vi "Change_state.vi"(7 "connect (T)":bool=TRUE, 10 "Z_HSwitch_state in":T2={"Write"=FALSE, "Z1_ind visu"=5, "Z1_ind_blinking"=FALSE, "Z_HSwitch_out"=FALSE, "Z_HSwitch_visible"=FALSE, "Z_HSwitch_disabled"=enum."Enabled"}, 11 "Z_Source":T1=enum."local disabled") -> (1 "reset_timer":bool, 2 "Z_HSwitch_state out":T2, 3 "Z1_ind_state":T3 items=["init", "not connect", "local disabled", "local hand", "set hand", "hand", "set auto", "auto", "dist"], 4 "load_timer":bool)   [LabVIEW 2019, in "Heating.lvlib"]
uses:
  Heating.lvlib
  ctl/Z_Hswitch/AutoButton_state.ctl
  ctl/Z_source.ctl
  ctl/Z_Hswitch/Z_Hswitch.xctl
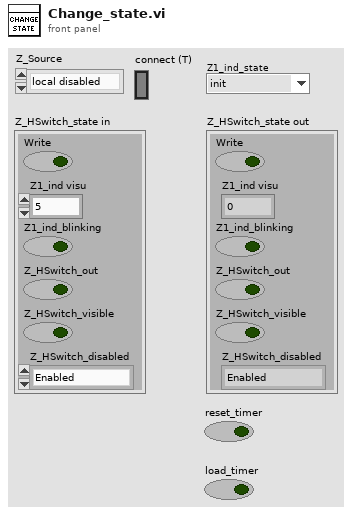
[diagram p1: front panel]
types:
  T1 = typedef "Heating.lvlib/Z_source.ctl" = enum8{"initialize", "local disabled", "local hand", "hand", "auto", "dist"}
  T2 = cluster{"Write":bool, "Z1_ind visu":u8, "Z1_ind_blinking":bool, "Z_HSwitch_out":bool, "Z_HSwitch_visible":bool, "Z_HSwitch_disabled":enum8{"Enabled", "Disabled", "Disabled and Grayed Out"}}
  T3 = typedef "Heating.lvlib/Z_Hswitch.xctl/AutoButton_state.ctl" = u16
  T4 = enum8{"Enabled", "Disabled", "Disabled and Grayed Out"}
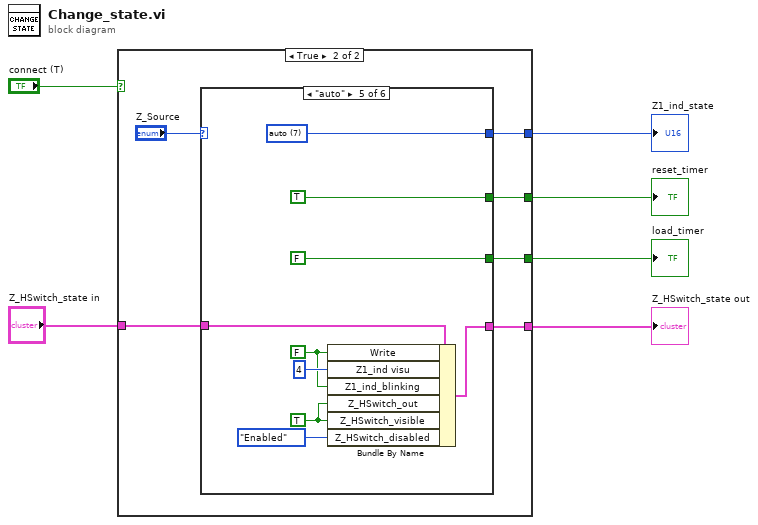
[diagram p0: block diagram]
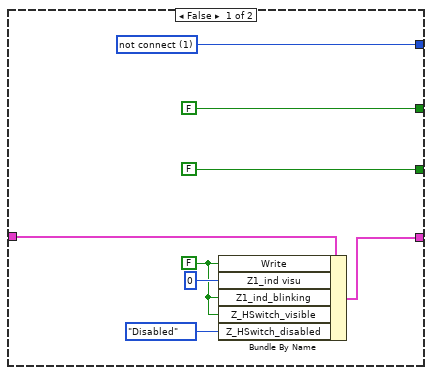
[diagram p2: hidden frame]
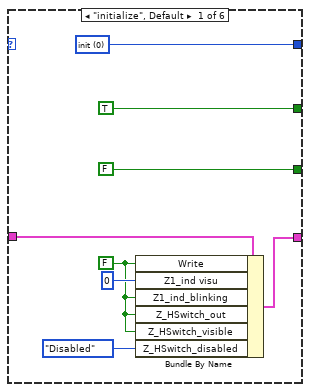
[diagram p3: hidden frame]
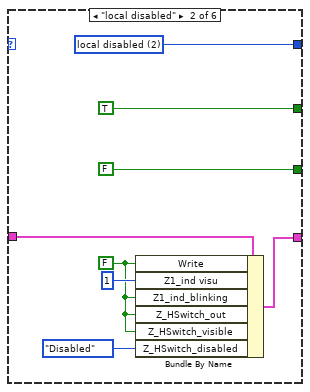
[diagram p4: hidden frame]
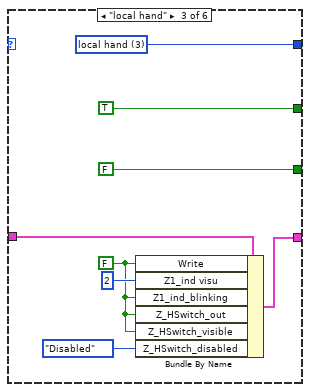
[diagram p5: hidden frame]
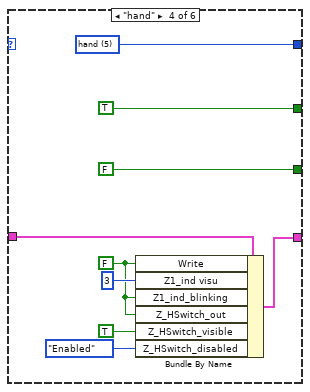
[diagram p6: hidden frame]
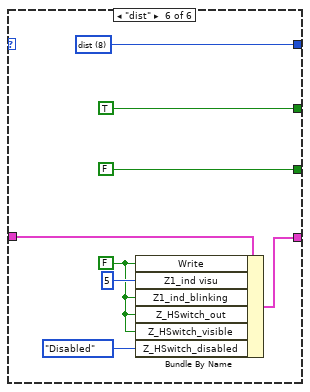
[diagram p7: hidden frame]
diagram:
  n1 = case shown="True" "connect (T)" {
    tunnel: "Z_HSwitch_state in" -> [w10 w20]
    tunnel: [w14 w18] -> w5
    tunnel: [FALSE ("Z_ASwitch") w17] -> w4
    tunnel: [FALSE ("Z_ASwitch") w16] -> w3
    tunnel: [w11 w15] -> w2
    frame False {
      w8 = FALSE ("Z_ASwitch")
      w14 = T3 1 items=["init", "not connect", "local disabled", "local hand", "set hand", "hand", "set auto", "auto", "dist"] ("Z1_State")
      n2 = Bundle By Name(cluster=w10, "Write"=w8, "Z1_ind visu"=u8 0, "Z1_ind_blinking"=w8, "Z_HSwitch_visible"=w8, "Z_HSwitch_disabled"=T4."Disabled" ("Disabled")) -> (w11:T2)
    }
    frame True {
      n3 = case shown="\"auto\"" "Z_Source" {
        tunnel: w20 -> [w26 w34 w42 w51 w60 w68]
        tunnel: [w25 w33 w41 w50 w59 w67] -> w18
        tunnel: [TRUE ("Z_ASwitch") TRUE ("Z_ASwitch") TRUE ("Z_ASwitch") TRUE ("Z_ASwitch") TRUE ("Z_ASwitch") TRUE ("Z_ASwitch")] -> w17
        tunnel: [FALSE ("Z_ASwitch") FALSE ("Z_ASwitch") FALSE ("Z_ASwitch") FALSE ("Z_ASwitch") FALSE ("Z_ASwitch") FALSE ("Z_ASwitch")] -> w16
        tunnel: [w22 w30 w38 w47 w56 w64] -> w15
        frame "initialize", Default {
          w21 = FALSE ("Z_ASwitch")
          w25 = T3 0 items=["init", "not connect", "local disabled", "local hand", "set hand", "hand", "set auto", "auto", "dist"] ("Z1_State")
          n4 = Bundle By Name(cluster=w26, "Write"=w21, "Z1_ind visu"=u8 0, "Z1_ind_blinking"=w21, "Z_HSwitch_out"=w21, "Z_HSwitch_visible"=w21, "Z_HSwitch_disabled"=T4."Disabled" ("Disabled")) -> (w22:T2)
        }
        frame "local disabled" {
          w29 = FALSE ("Z_ASwitch")
          w33 = T3 2 items=["init", "not connect", "local disabled", "local hand", "set hand", "hand", "set auto", "auto", "dist"] ("Z1_State")
          n5 = Bundle By Name(cluster=w34, "Write"=w29, "Z1_ind visu"=u8 1, "Z1_ind_blinking"=w29, "Z_HSwitch_out"=w29, "Z_HSwitch_visible"=w29, "Z_HSwitch_disabled"=T4."Disabled" ("Disabled")) -> (w30:T2)
        }
        frame "local hand" {
          w37 = FALSE ("Z_ASwitch")
          w41 = T3 3 items=["init", "not connect", "local disabled", "local hand", "set hand", "hand", "set auto", "auto", "dist"] ("Z1_State")
          n6 = Bundle By Name(cluster=w42, "Write"=w37, "Z1_ind visu"=u8 2, "Z1_ind_blinking"=w37, "Z_HSwitch_out"=w37, "Z_HSwitch_visible"=w37, "Z_HSwitch_disabled"=T4."Disabled" ("Disabled")) -> (w38:T2)
        }
        frame "hand" {
          w46 = FALSE ("Z_ASwitch")
          w50 = T3 5 items=["init", "not connect", "local disabled", "local hand", "set hand", "hand", "set auto", "auto", "dist"] ("Z1_State")
          n7 = Bundle By Name(cluster=w51, "Write"=w46, "Z1_ind visu"=u8 3, "Z1_ind_blinking"=w46, "Z_HSwitch_out"=w46, "Z_HSwitch_visible"=TRUE ("Z_ASwitch"), "Z_HSwitch_disabled"=T4."Enabled" ("Disabled")) -> (w47:T2)
        }
        frame "auto" {
          w54 = TRUE ("Z_ASwitch")
          w55 = FALSE ("Z_ASwitch")
          w59 = T3 7 items=["init", "not connect", "local disabled", "local hand", "set hand", "hand", "set auto", "auto", "dist"] ("Z1_State")
          n8 = Bundle By Name(cluster=w60, "Write"=w55, "Z1_ind visu"=u8 4, "Z1_ind_blinking"=w55, "Z_HSwitch_out"=w54, "Z_HSwitch_visible"=w54, "Z_HSwitch_disabled"=T4."Enabled" ("Disabled")) -> (w56:T2)
        }
        frame "dist" {
          w63 = FALSE ("Z_ASwitch")
          w67 = T3 8 items=["init", "not connect", "local disabled", "local hand", "set hand", "hand", "set auto", "auto", "dist"] ("Z1_State")
          n9 = Bundle By Name(cluster=w68, "Write"=w63, "Z1_ind visu"=u8 5, "Z1_ind_blinking"=w63, "Z_HSwitch_out"=w63, "Z_HSwitch_visible"=w63, "Z_HSwitch_disabled"=T4."Disabled" ("Disabled")) -> (w64:T2)
        }
      }
    }
  }
  "Z1_ind_state" <- w5
  "load_timer" <- w3
  "reset_timer" <- w4
  "Z_HSwitch_state out" <- w2
